vi "Tabor 5064 - Set Sine Phase (SubVI).vi"(6 "write_delay (ms)":u32=100, 7 "GPIB Address":string="4", 8 "error_in":errorcluster, 11 "phases (deg)":dbl[](array[numeric])) -> (0 "error_out":errorcluster)   [LabVIEW 2018]
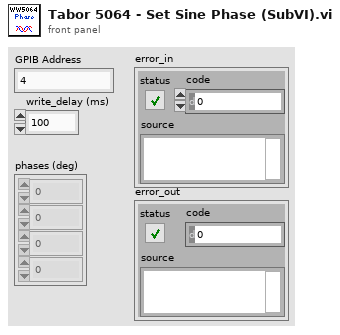
[diagram p1: front panel]
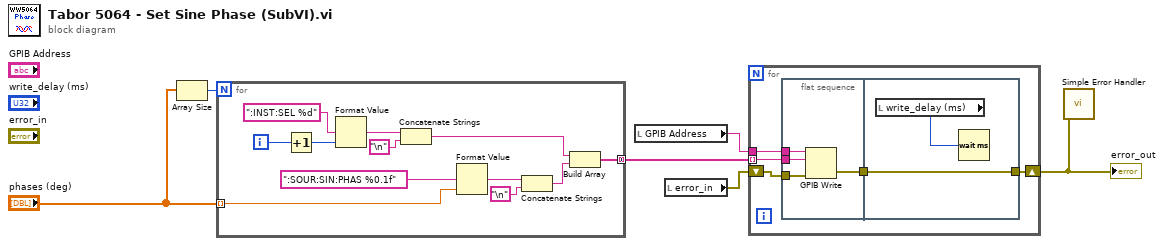
[diagram p0: block diagram]
diagram:
  n1 = Array Size(array="phases (deg)") -> (size(s)=w5:i32)
  n2 = for {
    N: w5 -> [_]
    tunnel: "phases (deg)" -> [w14] mode=indexing
    tunnel: [w9] -> w3 mode=concatenating
    i -> [w15]
    n3 = Increment(x=w15) -> (x+1=w16:i32)
    n4 = Format Value(format string=":INST:SEL %d", value (0)=w16) -> (output string=w11:string)  [unwired: 1 in]
    n5 = Concatenate Strings(w11, "\n") -> (w10:string)
    n6 = Format Value(format string=":SOUR:SIN:PHAS %0.1f", value (0)=w14) -> (output string=w8:string)  [unwired: 1 in]
    n7 = Concatenate Strings(w8, "\n") -> (w7:string)
    n8 = Build Array(w10, w7) -> (w9:string[])
  }
  n9 = local read "GPIB Address"() -> (w2:string)
  n10 = local read "error_in"() -> (w1:errorcluster)
  n11 = for {
    tunnel: w2 -> [w23]
    tunnel: w3 -> [w22] mode=indexing
    shift-right: [w21] -> w6
    shift-left: w1 -> [w20]
    n12 = flat-sequence {
      tunnel: w23 -> [w27]
      tunnel: w22 -> [w26]
      tunnel: w20 -> [w24]
      tunnel: [w25] -> w19
      tunnel: [w29] -> w21
      tunnel: w19 -> [w29]
      frame #0 {
        n13 = GPIB Write(0:w27, 1:w26, 3:w24) -> (6:w25:errorcluster)  [unwired: 2 in, 1 out]
      }
      frame #1 {
        n14 = local read "write_delay (ms)"() -> (w28:u32)
        n15 = Wait (ms)(milliseconds to wait=w28) -> ()  [unwired: 1 out]
      }
    }
  }
  "error_out" <- w6
  n16 = call <vilib>:"Simple Error Handler.vi"("error in (no error)"=w6) -> ()  [unwired: 4 in, 5 out]
